vi "lvpeak_close_camera.vi"(8 "error in (no error)":errorcluster, 11 "camera_id":u64) -> (0 "error out":errorcluster)   [LabVIEW 2024, in "Vision.lvlib"]
uses:
  Vision.lvlib
  bin/LVPeak.dll
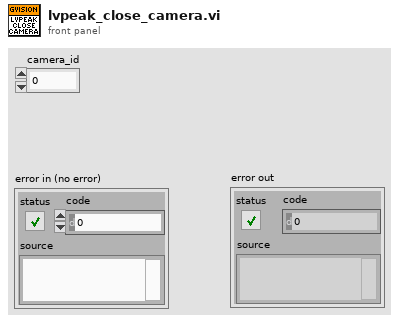
[diagram p1: front panel]
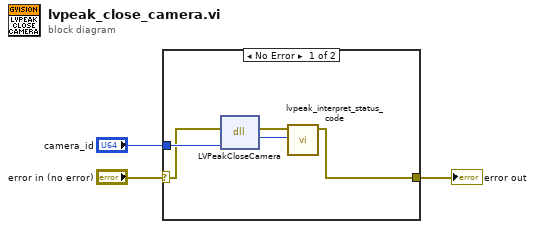
[diagram p0: block diagram]
diagram:
  n1 = case shown="No Error" "error in (no error)" {
    selector: "error in (no error)" -> [w5 w9]
    tunnel: [w4 w9] -> w2
    tunnel: "camera_id" -> [w6 _]
    frame No Error {
      n2 = dll-call lib="C:/Users/cfang/Desktop/nebraska-silicon-lab/pixel-gantry-control/Gantry/Shared Components/bin/LVPeak.dll" fn="LVPeakCloseCamera"(error in=w5, "camera_id"=w6) -> (error out=w8:errorcluster, "return type"=w7:i32)  [unwired: 3 in, 1 out]
      n3 = call "lvpeak_interpret_status_code.vi"("status_code"=w7, "error in (no error)"=w8) -> ("error out"=w4:errorcluster)  [unwired: 9 in]
    }
    frame Error {
    }
  }
  "error out" <- w2
